vi "Open system.vi"() -> (0 "error out":errorcluster caption="sortie d'erreur", 1 "Configuration data":T3, 2 "All Message Queue Cluster":T1, 3 "Notifiers":T2)   [LabVIEW 2013]
uses:
  Lib Data Config/Data Config.ctl
  Lib Notifier/Notifier.ctl
  Lib QMH/AllMessageQueue Cluster.ctl
  Lib QMH/Message Cluster.ctl
  Lib QMH/MessageQueues.lvlib
  Lib Notifier/Notifier.lvlib
  Lib Data Config/Data Configuration File.lvlib
panel:
  in  "entrée d'erreur":errorcluster
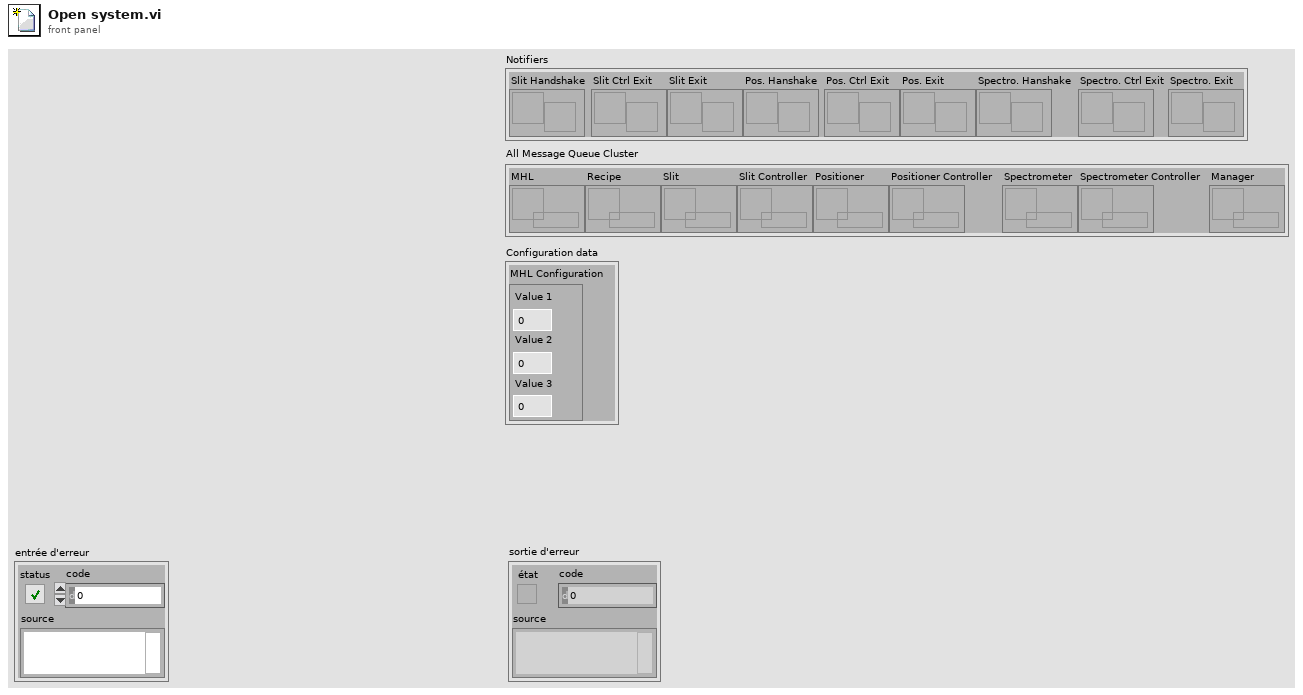
[diagram p1: front panel]
types:
  T1 = typedef "MessageQueues.lvlib/AllMessageQueue Cluster.ctl" = cluster{"MHL":refnum<queue>, "Recipe":refnum<queue>, "Slit":refnum<queue>, "Slit Controller":refnum<queue>, "Positioner":refnum<queue>, "Positioner Controller":refnum<queue>, "Spectrometer":refnum<queue>, "Spectrometer Controller":refnum<queue>, "Manager":refnum<queue>}
  T2 = typedef "Notifier.lvlib/Notifier.ctl" = cluster{"Slit Handshake":refnum<notifier>, "Slit Ctrl Exit":refnum<notifier>, "Slit Exit":refnum<notifier>, "Pos. Hanshake":refnum<notifier>, "Pos. Ctrl Exit":refnum<notifier>, "Pos. Exit":refnum<notifier>, "Spectro. Hanshake":refnum<notifier>, "Spectro. Ctrl Exit":refnum<notifier>, "Spectro. Exit":refnum<notifier>}
  T3 = typedef "Data Configuration File.lvlib/Data Config.ctl" = cluster{"MHL Configuration":cluster{"Value 1":dbl, "Value 2":dbl, "Value 3":dbl}}
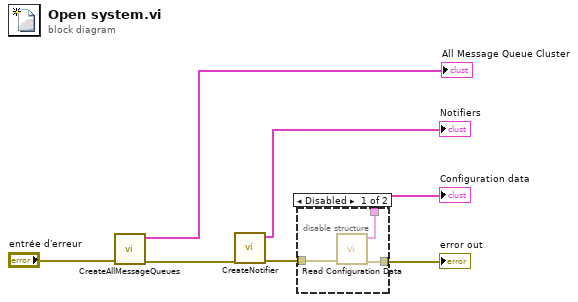
[diagram p0: block diagram]
diagram:
  n1 = call "CreateAllMessageQueues.vi"("entrée d'erreur"="entrée d'erreur") -> ("error out"=w6:errorcluster, "All Message Queue Cluster"=→"All Message Queue Cluster":T1)  [unwired: 9 in]
  n2 = call "CreateNotifier.vi"("entrée d'erreur (pas d'erreur)"=w6) -> ("sortie d'erreur"=w5:errorcluster, "Notifiers"=→"Notifiers":T2)  [unwired: 9 in]
  n3 = disable-structure shown="Disabled" {
    disable-tunnel: w5 -> [w10 w11]
    disable-tunnel: [w9 w11] -> w4
    disable-tunnel: [w8 _] -> w1
    frame Disabled {
      n4 = call "Read Configuration Data.vi"("error in (no error)"=w10) -> ("error out"=w9:errorcluster, "Configuration data"=w8:T3)  [unwired: 9 in]
    }
    frame Enabled {
    }
  }
  "error out" <- w4
  "Configuration data" <- w1
